vi "Start Config.vi"(8 "error in":errorcluster, 11 "PAS in":refnum<class "PAS.lvclass">) -> (0 "error out":errorcluster, 3 "PAS out":refnum<class "PAS.lvclass">)   [LabVIEW 2014, in "PAS.lvclass"]
doc: "Perform configuration of cells and data classes as well as switching and anything else that might not fit into the other config VIs. This VI can be used to set up a single cell with the default PAS Data Class, PAS Cell class, and a speaker switch setting of firing every 5 minutes for 1 second."
uses:
  PAS.lvclass
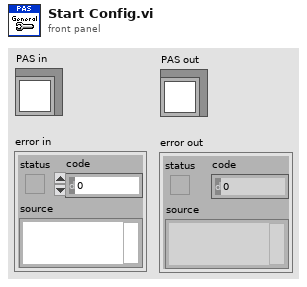
[diagram p1: front panel]
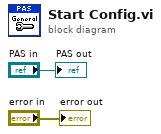
[diagram p0: block diagram]
diagram:
  "error out" <- "error in"
  "PAS out" <- "PAS in"
